vi "Error Query.vi"(4 "Expected read buffer":string, 6 "Last command":string, 7 "Ignore empty sequence? (T)":bool=TRUE, 8 "error in (no error)":errorcluster, 10 "Read buffer":string, 11 "VISA resource name":refnum<visa-resource-name>) -> (0 "error out":errorcluster, 3 "VISA resource name out":refnum<visa-resource-name>)   [LabVIEW 2020, in "QuPMXdriver.lvlib"]
doc: "Checks if expected read buffer is same as real read buffer (only if expected read buffer is not empty).\nChecks status byte and generate error if any.\nIgnore empty sequence: ignores device error \"No switching sequence\".\n\n<B>Note:</B>\nThis VI is called automatically by most driver VIs so it is not usually necessary to call this in an application."
uses:
  QuPMXdriver.lvlib
  <vilib>/ErrorRing/Error Ring.xnode
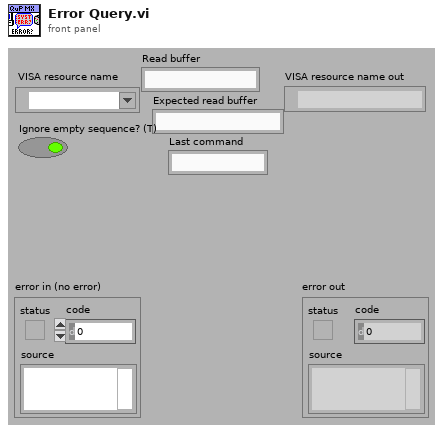
[diagram p1: front panel]
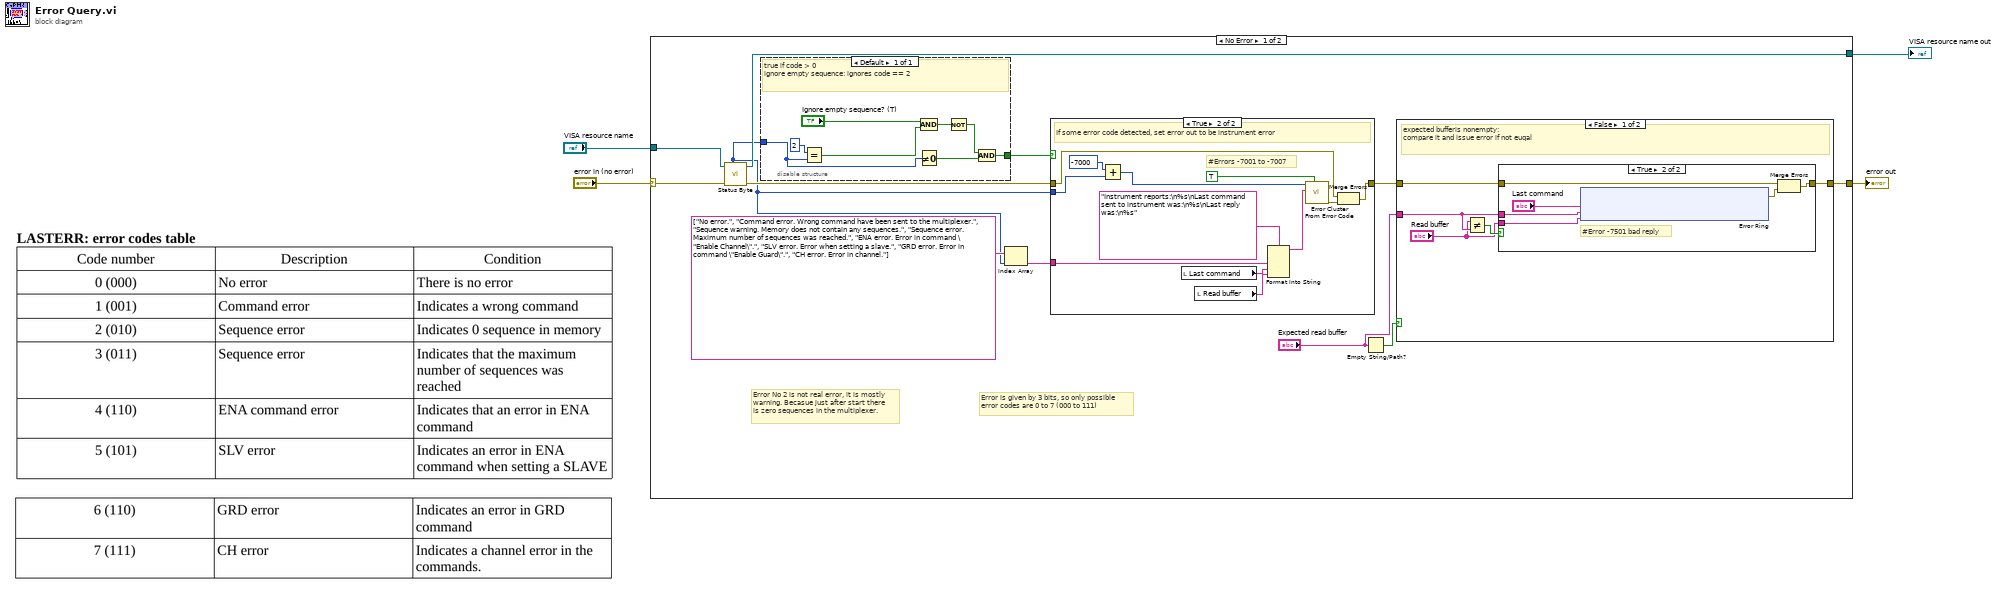
[diagram p0: block diagram]
diagram:
  n1 = case shown="No Error" "error in (no error)" {
    selector: "error in (no error)" -> [w7 w60]
    tunnel: [w15 w61] -> w4
    tunnel: "VISA resource name" -> [w16 w61]
    tunnel: [w6 w60] -> w3
    frame No Error {
      # "Error is given by 3 bits, so only possible\nerror codes are 0 to 7 (000 to 111)"
      # "Error No 2 is not real error, it is mostly\nwarning. Becasue just after start there\nis zero sequences in the multiplexer."
      n2 = call "Status Byte.vi"("error in (no error)"=w7, "VISA resource name"=w16) -> ("error out"=w12:errorcluster, "VISA resource name out"=w15:refnum<visa-resource-name>, "Error number"=w8:i8)  [unwired: 2 in, 5 out]
      n3 = disable-structure shown="Default" {
        disable-tunnel: [w23] -> w11
        disable-tunnel: w8 -> [w17]
        frame Enabled {
          # "true if code > 0\nignore empty sequence: ignores code == 2"
          n4 = Equal?(x=i8 2, y=w17) -> (x = y?=w20:bool)
          n5 = Not Equal To 0?(x=w17) -> (x != 0?=w24:bool)
          n6 = Compound Arithmetic op=AND("Ignore empty sequence? (T)", w20) -> (w19:bool)
          n7 = Not(x=w19) -> (.not. x?=w18:bool)
          n8 = Compound Arithmetic op=AND(w18, w24) -> (w23:bool)
        }
      }
      n9 = Index Array(array=string[] ["No error.", "Command error. Wrong command have been sent to the multiplexer.", "Sequence warning. Memory does not contain any sequences.", "Sequence error. Maximum number of sequences was reached.", "ENA error. Error in command \"Enable Channel\".", "SLV error. Error when setting a slave.", "GRD error. Error in command \"Enable Guard\".", "CH error. Error in channel."], index=w8) -> (element=w13:string)
      n10 = case shown="True" w11 {
        tunnel: w13 -> [_ w58]
        tunnel: [w47 w48] -> w5
        tunnel: w12 -> [w47 w50]
        tunnel: w8 -> [_ w52]
        frame False {
        }
        frame True {
          # "#Errors -7001 to -7007"
          # "If some error code detected, set error out to be instrument error"
          n11 = Add(x=-7000 ("Code"), y=w52) -> (x+y=w51:i32)
          n12 = local read "Last command"() -> (w55:string)
          n13 = local read "Read buffer"() -> (w56:string)
          n14 = Format Into String(format string="Instrument reports:\n%s\nLast command sent to instrument was:\n%s\nLast reply was:\n%s", w58, w55, w56) -> (resulting string=w54:string)  [unwired: 2 in, 1 out]
          n15 = call <vilib>:"Error Cluster From Error Code.vi"("show call chain? (False)"=TRUE, "error message (\"\")"=w54, "error code (0)"=w51) -> ("error out"=w49:errorcluster)  [unwired: 6 in]
          n16 = Merge Errors(w50, w49) -> (w48:errorcluster)
        }
      }
      n17 = Empty String/Path?(string/path="Expected read buffer") -> (empty?=w9:bool)
      n18 = case shown="False" w9 {
        tunnel: w5 -> [w28 w46]
        tunnel: [w27 w46] -> w6
        tunnel: "Expected read buffer" -> [w26 _]
        frame False {
          # "expected bufferis nonempty:\ncompare it and issue error if not euqal"
          n19 = Not Equal?(x="Read buffer", y=w26) -> (x != y?=w29:bool)
          n20 = case shown="True" w29 {
            tunnel: w28 -> [w30 w36]
            tunnel: [w30 w35] -> w27
            tunnel: w26 -> [_ w32]
            tunnel: "Read buffer" -> [_ w31]
            frame False {
            }
            frame True {
              # "#Error -7501 bad reply"
              n21 = xnode "Error Ring"("parameter 0"="Last command", "parameter 1"=w32, "parameter 2"=w31) -> ("error out"=w34:errorcluster)
              n22 = Merge Errors(w36, w34) -> (w35:errorcluster)
            }
          }
        }
        frame True {
        }
      }
    }
    frame Error {
    }
  }
  "VISA resource name out" <- w4
  "error out" <- w3
